vi "New_files_queue.vi"(10 "filenames new":string[](array[string]), 11 "filenames old":string[](array[string])) -> (3 "Filenames":string[](array[string]))   [LabVIEW 2019]
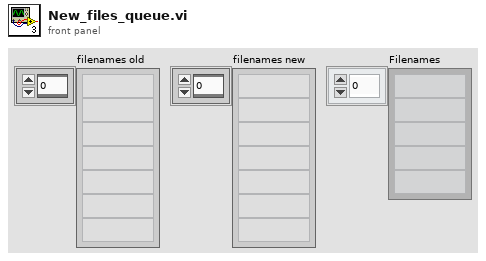
[diagram p1: front panel]
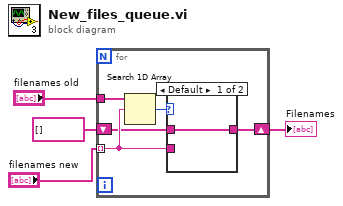
[diagram p0: block diagram]
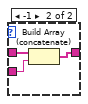
[diagram p2: hidden frame]
diagram:
  n1 = for {
    tunnel: "filenames new" -> [w8] mode=indexing
    tunnel: "filenames old" -> [w7]
    shift-right: [w6] -> w2
    shift-left: string[] [] -> [w5]
    n2 = Search 1D Array(1D array=w7, element=w8) -> (index of element=w9:i32)  [unwired: 1 in]
    n3 = case shown="Default" w9 {
      tunnel: w8 -> [_ w13]
      tunnel: [w10 w12] -> w6
      tunnel: w5 -> [w10 w11]
      frame Default {
      }
      frame -1 {
        n4 = Build Array (concatenate)(w11, w13) -> (w12:string[])
      }
    }
  }
  "Filenames" <- w2
